vi "Subvi pixel sync.vi"(2 "DO channel":refnum<k21>="Connector0/DIO5", 10 "Memory label":refnum<k21>="Pixel sync buffer") -> ()   [LabVIEW 2017]
uses:
  <vilib>/rvi/Emulation/niFpgaSctlEmulationGetInTimedLoop.vi
  <vilib>/rvi/DataTransferAndStorage/Container/Common/niFpgaContainerExecOnDevCompGetState.vi
  <vilib>/rvi/Emulation/niFpgaEmulationIsFPGAContextNoSignature.vi
  <vilib>/rvi/DataTransferAndStorage/Container/Common/niFpgaContainerGetUniqueNameForEmu.vi
  <vilib>/rvi/Emulation/niFpgaProcessEmulError.vi
  <vilib>/rvi/errors/nirviReportUnexpectedCaseInternalError (U32).vi
  <vilib>/rvi/Memory/Memory_Emulation/niFpgaMemoryEmulationCacheClearOnFirstRun.vi
  <vilib>/rvi/Memory/Memory_Emulation/nirvimemoryEmulationManagerCache_MakeExclusive.vi
  <vilib>/rvi/Memory/Memory_Emulation/niFpgaMemoryEmulationValidateCache.vi
  <vilib>/rvi/Memory/Memory_Emulation/nirvimemoryEmulationManagerCache_InsertValue.vi
  <vilib>/Utility/error.llb/Clear Errors.vi
  <vilib>/rvi/Memory/Memory_Emulation/nirvimemoryEmulationManagerCache_ReleaseExclusive.vi
  <vilib>/rvi/Memory/Memory_Emulation/nirvimemoryEmulationManagerCache_GetValue.vi
  <vilib>/rvi/Memory/Memory_Emulation/nirvimemoryEmulationManagerCache_SetValue.vi
  <vilib>/rvi/Emulation/niFpgaSctlEmulationResourceMgr.vi
  GV Npix.vi
  GV pixel sync.vi
  <vilib>/rvi/eio/common/nirviEmuTemplateMethod_errors.vi
  <vilib>/rvi/DataTransferAndStorage/Container/XNode/niFpgaContainer.xnode
  <vilib>/rvi/Memory/Memory_Emulation/niFpgaMemoryEmulationRefIn.vi
  <vilib>/eio/EIONode/EIONode.xnode
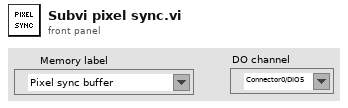
[diagram p1: front panel]
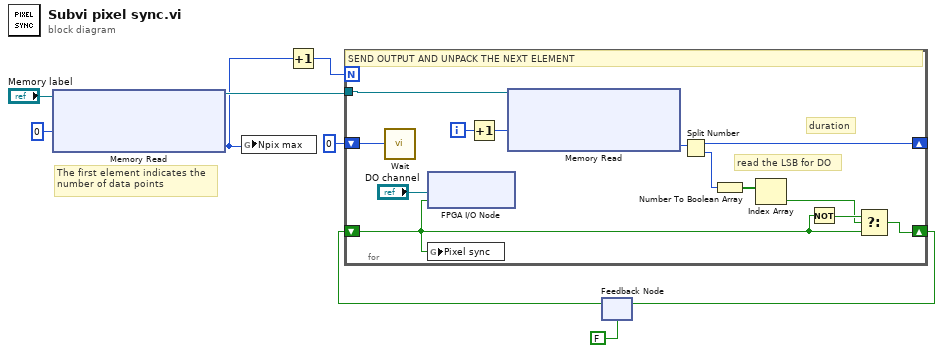
[diagram p0: block diagram]
diagram:
  # "The first element indicates the\nnumber of data points"
  n1 = xnode ("Memory Read")("Address"=u32 0, "Memory In"="Memory label") -> ("Data"=w1:u32, "Memory Out"=w9:refnum<k21>)
  n2 = global write "GV Npix.vi" "Npix max"(w1) -> ()
  n3 = Increment(x=w1) -> (x+1=w8:u32)
  n4 = feedback #1(FALSE) -> (w3:bool)
  n5 = for {
    N: w8 -> [_]
    shift-right: [w11] -> w4
    shift-left: w3 -> [w10]
    shift-right: [w21] -> _
    shift-left: u16 0 -> [w20]
    tunnel: w9 -> [w17]
    i -> [w19]
    # "read the LSB for DO"
    # "duration"
    # "SEND OUTPUT AND UNPACK THE NEXT ELEMENT"
    n6 = call "Wait"("Count(Ticks)"=w20) -> ()  [unwired: 1 out]
    n7 = xnode "FPGA I/O Node"("I/O Item"=w10, "FPGA I/O In"="DO channel") -> ()  [unwired: 1 out]
    n8 = global write "GV pixel sync.vi" "Pixel sync"(w10) -> ()
    n9 = Increment(x=w19) -> (x+1=w18:i32)
    n10 = xnode ("Memory Read")("Address"=w18, "Memory In"=w17) -> ("Data"=w22:u32)  [unwired: 1 out]
    n11 = Split Number(x=w22) -> (hi(x)=w21:u16, lo(x)=w14:u16)
    n12 = Number To Boolean Array(number=w14) -> (Boolean array=w15:bool[])
    n13 = Index Array(array=w15) -> (element=w12:bool)  [unwired: 1 in]
    n14 = Not(x=w10) -> (.not. x?=w13:bool)
    n15 = Select(t=w13, s=w12, f=w10) -> (s? t:f=w11:bool)
  }
  n16 = feedback-in #1(w4) -> ()
